vi "Test shm get Event simulation Mode LV.vi"(8 "error in (no error)":errorcluster, 11 "logevent_simulationMode_Ctl":cluster{"mode":i32, "priority":i32}) -> (0 "error out":errorcluster, 2 "function return":i32, 3 "logevent_simulationMode_Ctl out":cluster{"mode":i32, "priority":i32})   [LabVIEW 2018, in "SALLV_Test.lvlib"]
doc: "int Test_shm_getEvent_simulationModeLV(Test_logevent_simulationModeLV *logevent_simulationMode_Ctl );"
uses:
  SALLV_Test.lvlib
  SALLV_Test.so
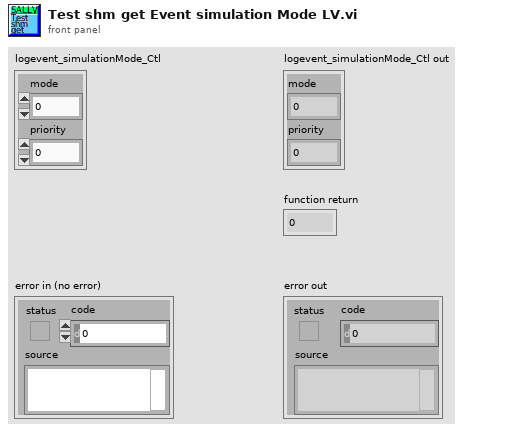
[diagram p1: front panel]
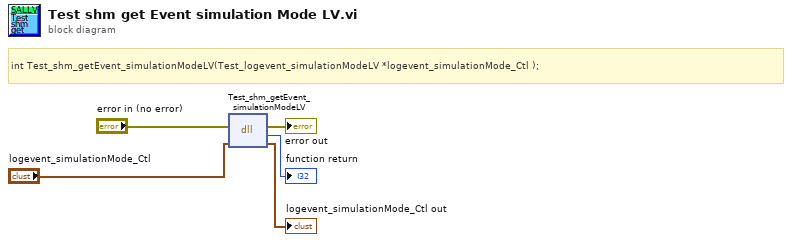
[diagram p0: block diagram]
diagram:
  # "int Test_shm_getEvent_simulationModeLV(Test_logevent_simulationModeLV *logevent_simulationMode_Ctl );"
  n1 = dll-call lib="home/ttsai/Documents/salLabVIEWtestData/SALLV_Test.*" fn="Test_shm_getEvent_simulationModeLV"(error in="error in (no error)", "logevent_simulationMode_Ctl"="logevent_simulationMode_Ctl") -> (error out=→"error out":errorcluster, →"function return":i32, "logevent_simulationMode_Ctl"=→"logevent_simulationMode_Ctl out":cluster{"mode":i32, "priority":i32})  [unwired: 2 in, 1 out]
